vi "BMA Controller(No Promp).vi"() -> ()   [LabVIEW 2010]
uses:
  SubVIs/FP Buttons.llb/Login Button__FP.ctl
  SubVIs/FP Buttons.llb/Diagnose Button__FP.ctl
  SubVIs/FP Buttons.llb/Exchange Button__FP.ctl
  SubVIs/FP Buttons.llb/Comments Button__FP.ctl
  SubVIs/Front Panel.llb/Reset.ctl
  SubVIs/General.llb/Time Control(System).ctl
  SubVIs/Front Panel.llb/Add Recipe__FP-BMA.ctl
  SubVIs/Front Panel.llb/Delete Recipe__FP-BMA.ctl
  SubVIs/Front Panel.llb/Define Recipe__FP-BMA.ctl
  SubVIs/Front Panel.llb/Operation__FP-BMA.ctl
  SubVIs/Front Panel.llb/Warnings__FP-BMA.ctl
  SubVIs/Front Panel.llb/Input__FP-BMA.ctl
  SubVIs/Front Panel.llb/Output__FP-BMA.ctl
  SubVIs/Front Panel.llb/PID Sets__FP-BMA.ctl
  SubVIs/Front Panel.llb/Cascade__FP-BMA.ctl
  SubVIs/Front Panel.llb/Current Step__FP-BMA.ctl
  SubVIs/Data Communication.llb/Plot Settings__DC-BMA.ctl
  SubVIs/FP Buttons.llb/Table Button(FTF)__FP.ctl
  SubVIs/FP Buttons.llb/Try Button__FP.ctl
  SubVIs/FP Buttons.llb/Print Button__FP.ctl
  SubVIs/FP Buttons.llb/Exit__FP.ctl
  SubVIs/Structure.llb/Queue Operation Mode__STR.ctl
  SubVIs/Structure.llb/Queues__STR.ctl
  SubVIs/Controller Communication.llb/F4 Controller Input Data Global Function Enumi.ctl
panel:
  out "Comm Status":string
  out "Exec Status":string
  in  "DataExchange":T1
  in  "Diagnose Comm":T2
  in  "Recipe":T3
  in  "Graph View":T4
  in  "EventLog":T5
  in  "Print":T6
  in  "Exit":T7
  in  "Login":T8
  in  "Tab":T9(tab)=enum."控制F4数据交换"
  in  "COM Diags":i32(listbox)
  in  "Reset Statistics":T10
  in  "Time Elapsed":string
  in  "Time Window":i32 caption="时间窗"
  in  "Time Schedule":T11(ring)
  in  "Modify":T12
  in  "Delete":T13
  in  "Add":T14
  in  "Recipe Name":u16(ring) caption="Recipe名称"
  in  "Recipe Start Time":T15 format="%<%.3X %x>T"
  in  "Calenda Schedule":i32(listbox)
  in  "Schedule Strings":string="2009-04-30 时间表"
  out "Event Strings":string
  in  "Plot Scroll":i32(c297)
  in  "Plot Settings":T16[](array[typedef]) caption="曲线设置"
  out "Trend Plot":waveform(dbl)(graph)
  in  "开始时间":T15 format="%<%.3X %x>T"
  in  "Duration":cluster{"Days":dbl, "Hrs":dbl, "Mins":dbl} caption="持续时间"
  in  "F4 Operation":T24={"operation"=TRUE, "Alarms"=FALSE, "Inputs"=FALSE, "Outputs"=FALSE, "PID Sets"=FALSE, "cascade"=FALSE, "Current Step"=FALSE} caption="F4操作"
  # "环境试验箱控制系统"
  # "重置后的时间消耗"
  # "估计时间窗"
  # "设置recipe开始时间"
  # "设置Recipe名称"
  # "时间表"
  # "显示   控制器                参数类型                 参数                    索引                    轴"
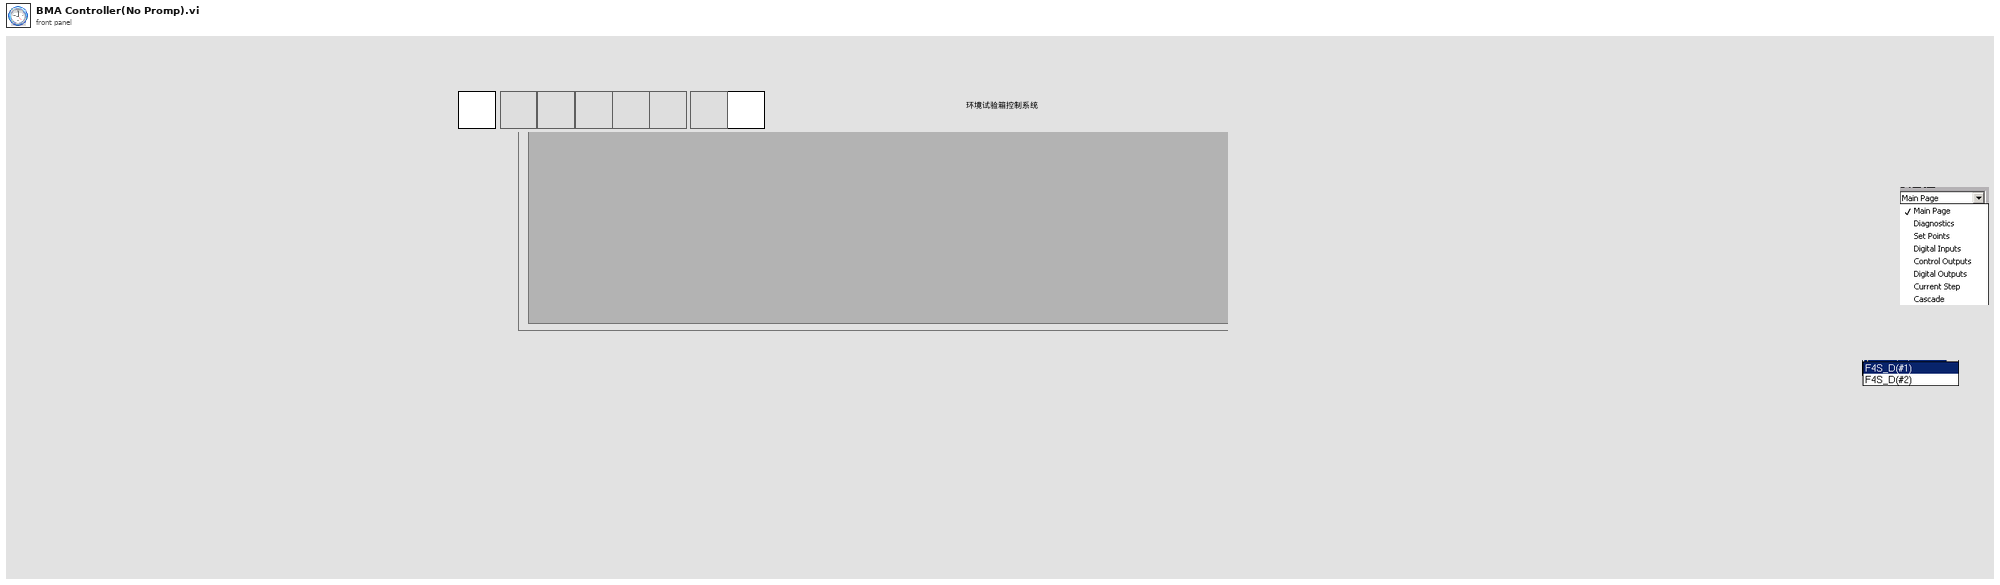
[diagram p1: front panel]
types:
  T1 = typedef "Try Button__FP.ctl" = bool
  T2 = typedef "Diagnose Button__FP.ctl" = bool
  T3 = typedef "Exchange Button__FP.ctl" = bool
  T4 = typedef "Table Button(FTF)__FP.ctl" = bool
  T5 = typedef "Comments Button__FP.ctl" = bool
  T6 = typedef "Print Button__FP.ctl" = bool
  T7 = typedef "Exit__FP.ctl" = bool
  T8 = typedef "Login Button__FP.ctl" = bool
  T9 = enum32{"通信诊断", "设置时间信息", "查看事件记录", "查看趋势图", "控制F4数据交换"}
  T10 = typedef "Reset.ctl" = bool
  T11 = enum16{"仅一次", "每隔数天", "每一天", "每个工作日", "每个周末", "每个月中的一天"}
  T12 = typedef "Define Recipe__FP-BMA.ctl" = bool
  T13 = typedef "Delete Recipe__FP-BMA.ctl" = bool
  T14 = typedef "Add Recipe__FP-BMA.ctl" = bool
  T15 = typedef "Time Control(System).ctl" = timestamp
  T16 = typedef "Plot Settings__DC-BMA.ctl" = cluster{"Show?":bool, "Controller Type":enum16{"F4S_D(#1)", "F4S_D(#2)"}, "Parameter":enum16{"主要页面", "诊断", "设置点", "数字输入", "控制输出", "数字输出", "当前步骤", "Cascade"}, "Parameter":enum16{"冷端补偿1", "冷端补偿2"}, "索引":enum16{"F4S_D(#1)"}, "Axis":string}
  T17 = typedef "Operation__FP-BMA.ctl" = bool
  T18 = typedef "Warnings__FP-BMA.ctl" = bool
  T19 = typedef "Input__FP-BMA.ctl" = bool
  T20 = typedef "Output__FP-BMA.ctl" = bool
  T21 = typedef "PID Sets__FP-BMA.ctl" = bool
  T22 = typedef "Cascade__FP-BMA.ctl" = bool
  T23 = typedef "Current Step__FP-BMA.ctl" = bool
  T24 = cluster{"operation":T17, "Alarms":T18, "Inputs":T19, "Outputs":T20, "PID Sets":T21, "cascade":T22, "Current Step":T23}
  T25 = typedef "Queue Operation Mode__STR.ctl" = enum16{"Noop", "Send Main", "Send Process", "Flush", "Destroy"}
  T26 = typedef "Queues__STR.ctl" = cluster{"main":T27, "process bar":T27}
  T27 = typedef "Queue RefNum" = refnum<k1>
  T28 = cluster{"[0]":bool, "[1]":bool, "[2]":bool, "[3]":bool, "[4]":bool, "[5]":bool, "[6]":bool}
  T29 = enum32{"Invalid", "Standard", "Closed", "Hidden", "Minimized", "Maximized"}
  T30 = enum32{"invalid app kind", "Development System", "Run Time System", "Student Edition", "Embedded LabVIEW", "Evaluation", "Custom"}
  T31 = typedef "F4 Controller Input Data Global Function Enumi.ctl" = enum16{"保存数据", "读取数据", "主程序状态写入", "主程序状态读取"}
  T32 = cluster{"Core":cluster{"Current VI Reference":refnum<vi>, "Close Panel on Exit?":bool}, "queues":T26, "Menu Refnum":refnum<k9>, "button":refnum<vi>[], "Tab":enum32{"通信诊断", "设置时间信息", "查看事件记录", "查看趋势图", "控制F4数据交换"}}
  T33 = cluster{"Current VI Reference":refnum<vi>, "Close Panel on Exit?":bool}
  T34 = typedef "Path InitPaths__FS.ctl" = cluster{"Ctrller CFG":path, "INI":path, "Profile":path, "EventLog":path, "Data":path}
  T35 = typedef "Controller Configuration__CHC.ctl" = cluster{"Ctrller Type":T36, "Ctrller Name":string, "Ctrller Addr":string, "Server IP":string, "Conn Result":string, "Port":string, "Baud":dbl}
  T36 = typedef "Controller Configuration__Ctrller Type.ctl" = enum16{"F4S/D", "Synergy"}
  T37 = typedef "Login Info__BMA-ULR.ctl" = cluster{"status":bool, "account":u16, "user":string}
  T38 = cluster{"Plot Settings":refnum<vi>, "Plot Scroll":refnum<vi>}
  T39 = typedef "Path InitDynamicVIsPaths__FS.ctl" = cluster{"F4 Operation":path, "F4 Alarms":path, "F4 Inputs":path, "F4 Outputs":path, "F4 PID Sets":path, "F4 Cascade":path, "F4 Current Step":path, "Profile SubPanel":path, "Profile Editor":path, "MainVI":path, "Profile Control":path, "Synergy Control":path, "Driver Server":path}
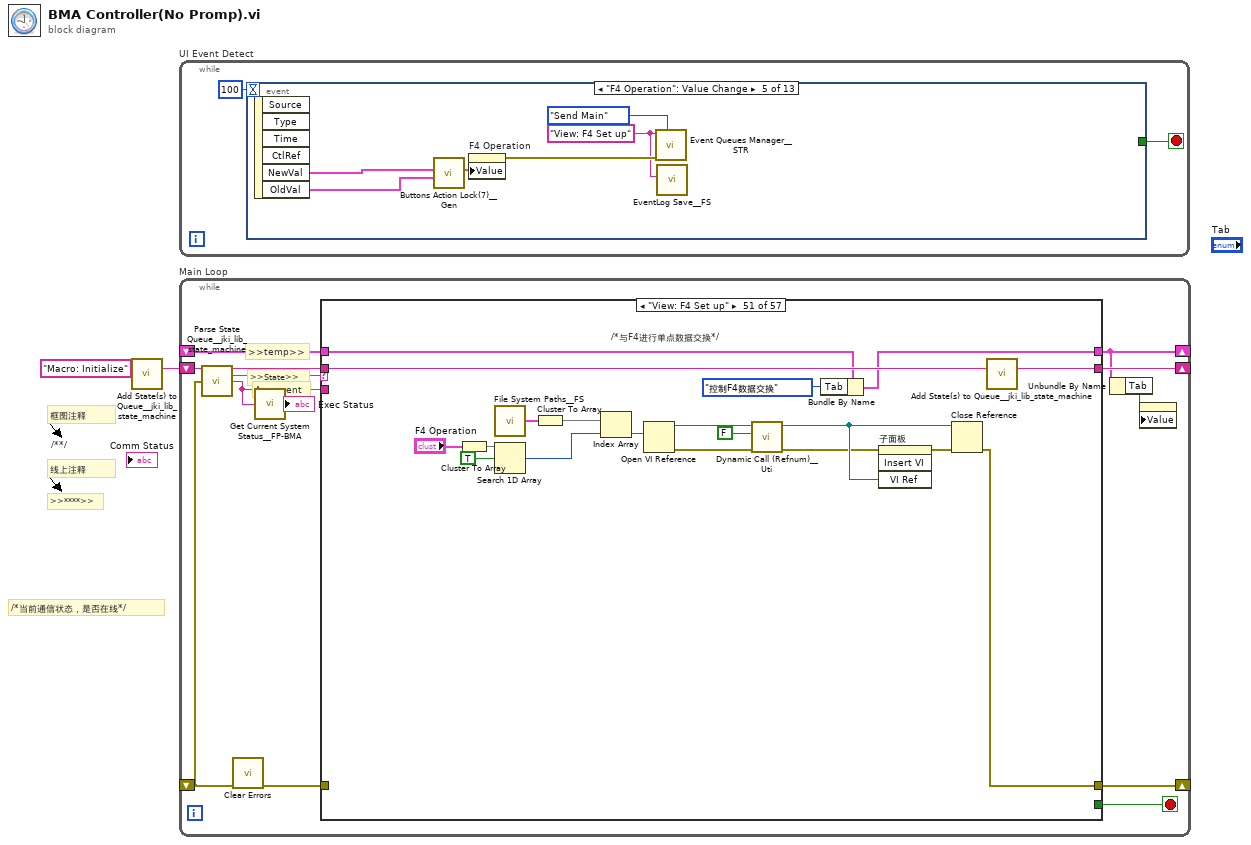
[diagram p0: block diagram]
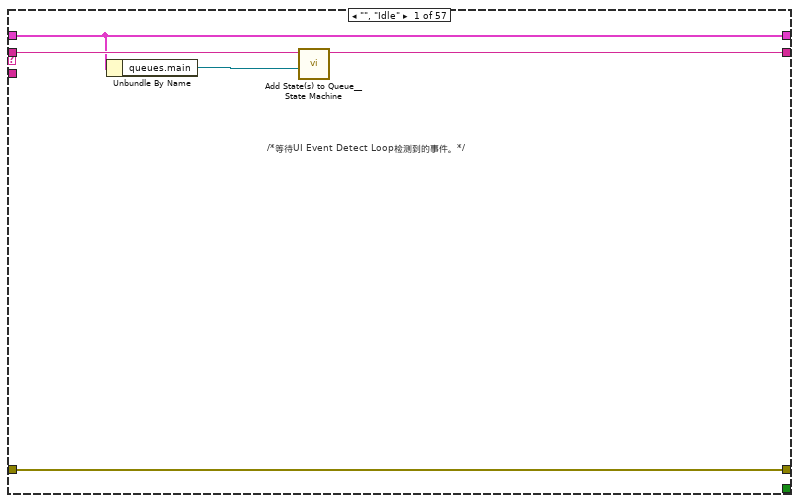
[diagram p2: hidden frame]
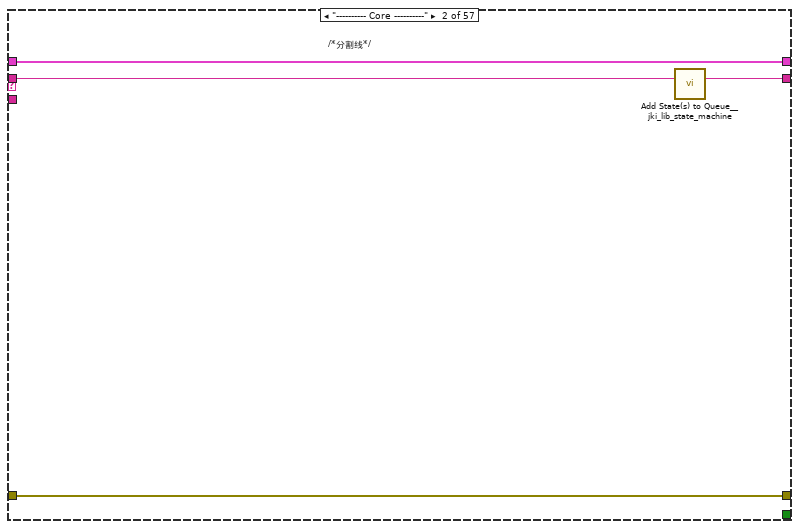
[diagram p3: hidden frame]
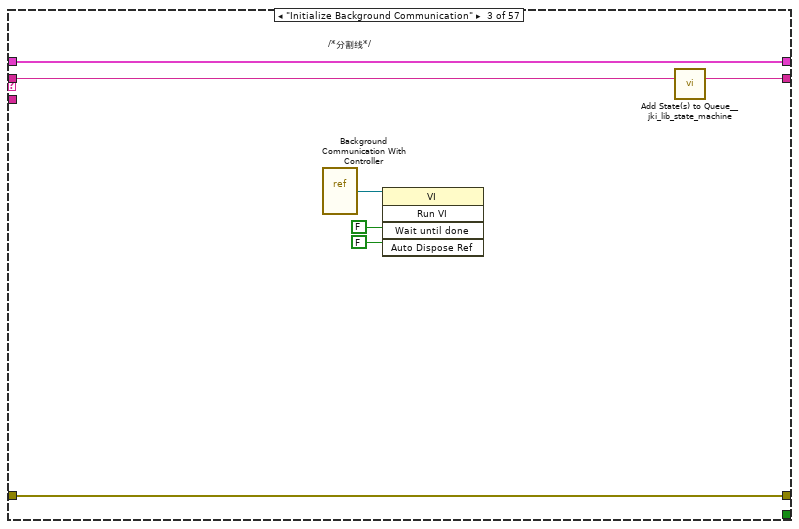
[diagram p4: hidden frame]
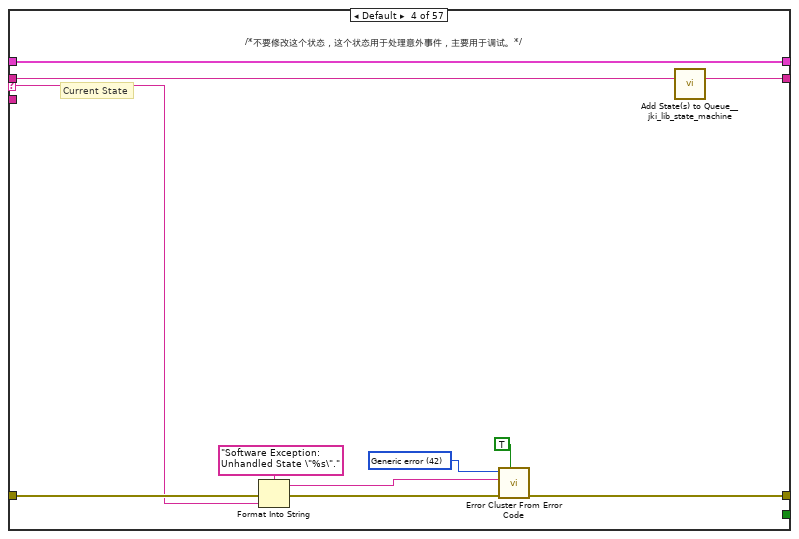
[diagram p5: hidden frame]
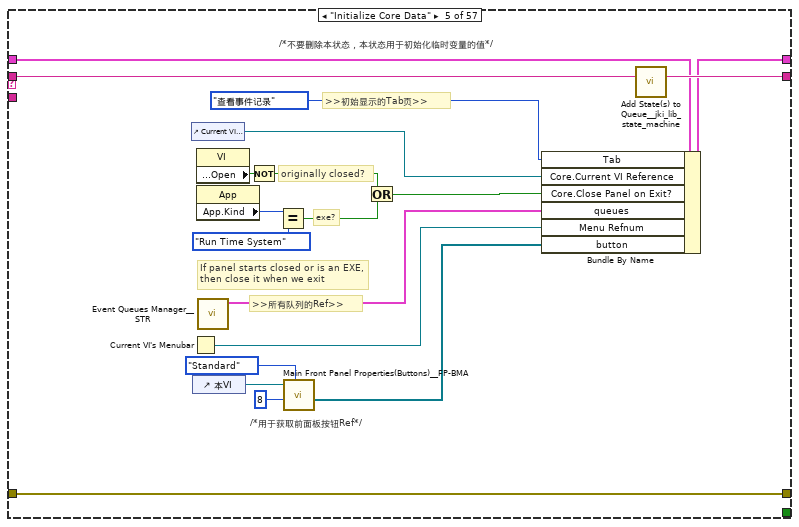
[diagram p6: hidden frame]
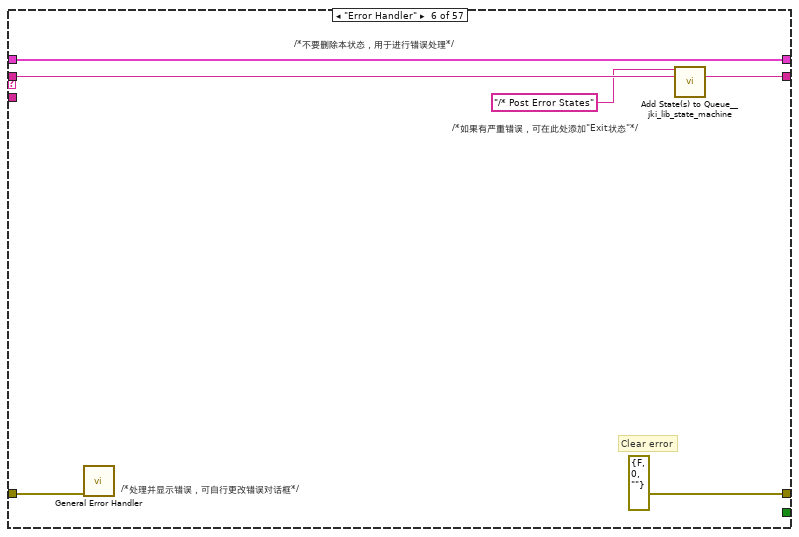
[diagram p7: hidden frame]
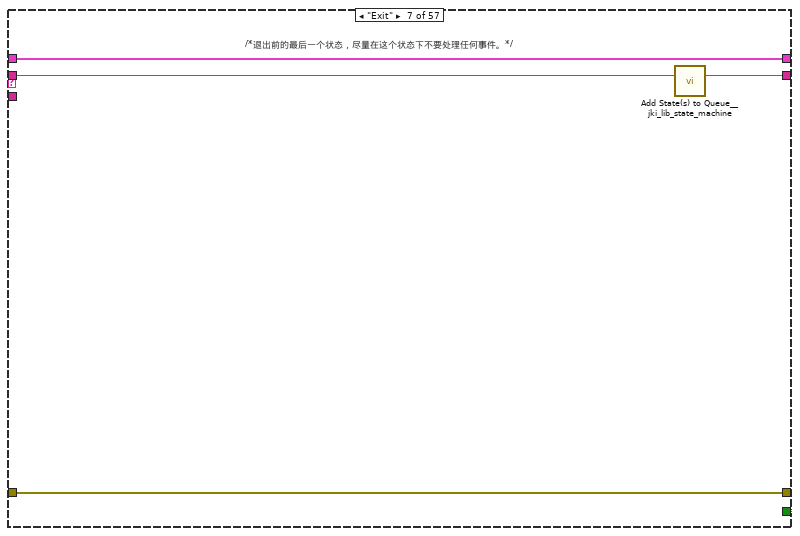
[diagram p8: hidden frame]
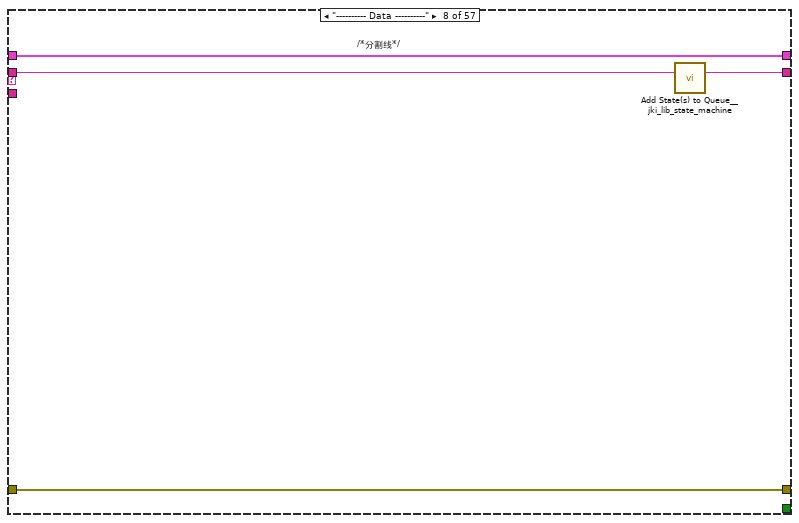
[diagram p9: hidden frame]
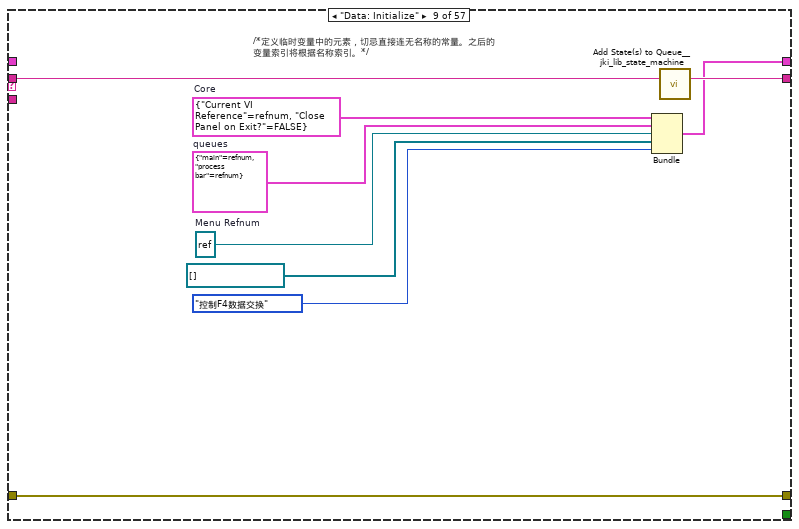
[diagram p10: hidden frame]
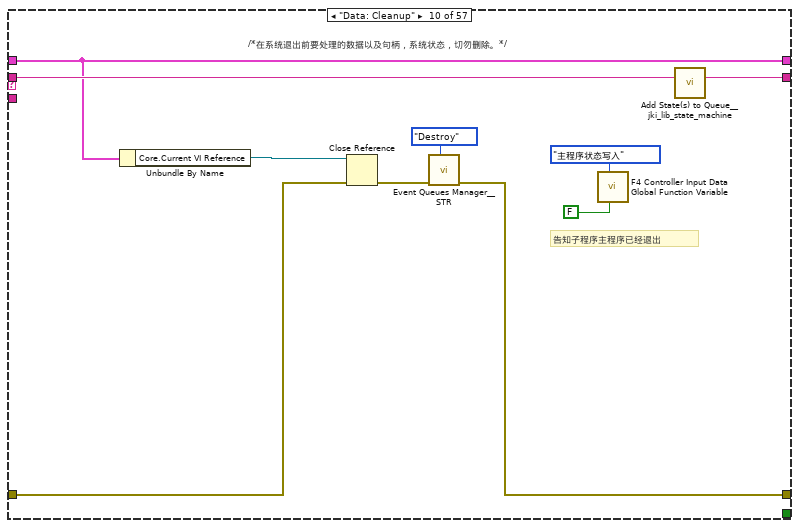
[diagram p11: hidden frame]
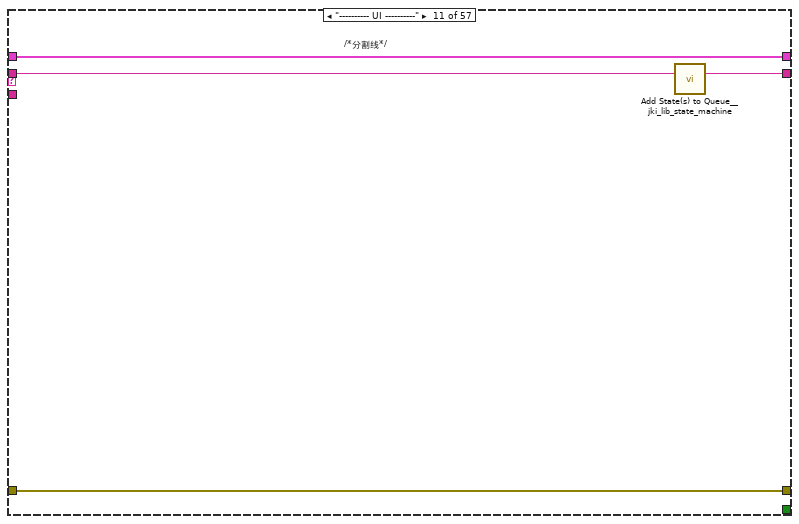
[diagram p12: hidden frame]
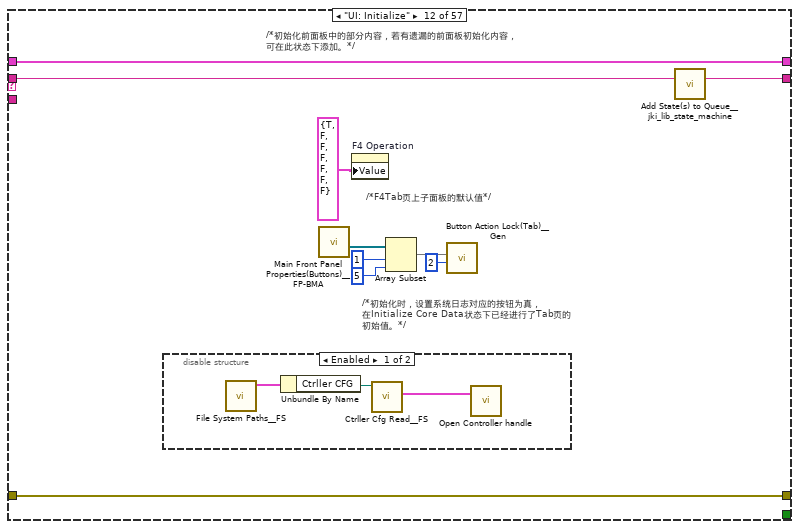
[diagram p13: hidden frame]
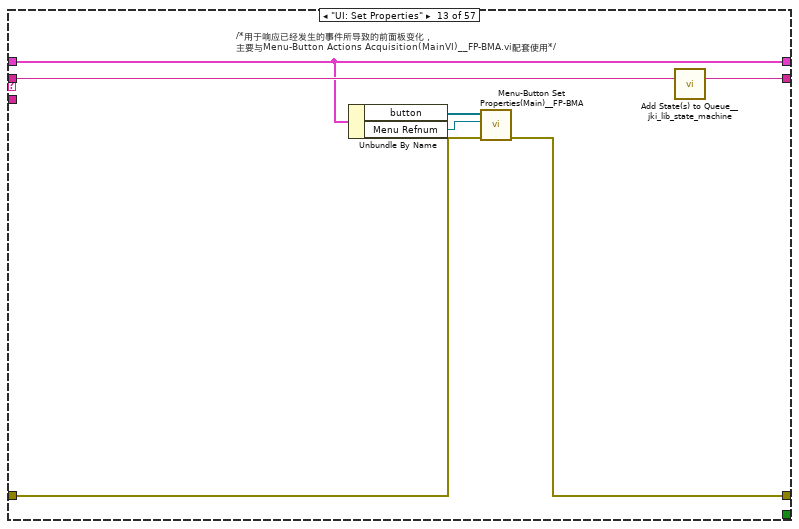
[diagram p15: hidden frame]
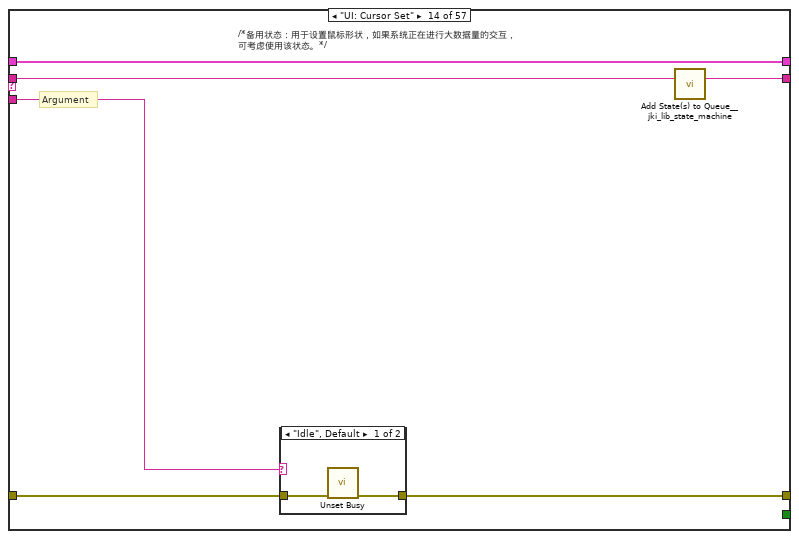
[diagram p16: hidden frame]
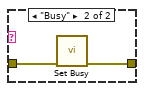
[diagram p17: hidden frame]
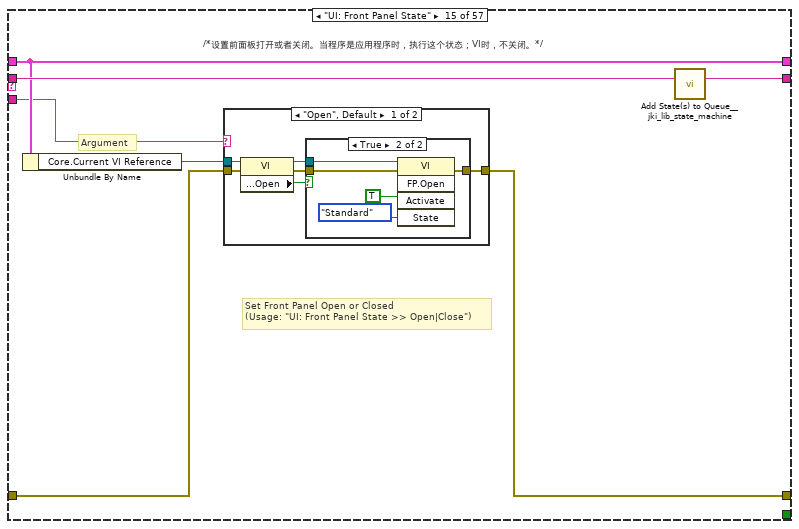
[diagram p18: hidden frame]
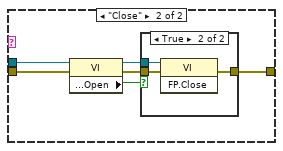
[diagram p20: hidden frame]
diagram:
  # "/**/"
  # "框图注释"
  # "线上注释"
  # ">>****>>"
  # "/*当前通信状态，是否在线*/"
  n1 = call "Add State(s) to Queue__jki_lib_state_machine.vi"("State(s) in (\"\")"="Macro: Initialize") -> ("States Out"=w1:string)  [unwired: 14 in]
  n2 = while "UI Event Detect" {
    stop <- w3 stop-if-true
    n3 = event shown="[4] \"F4 Operation\": Value Change" {
      selector: _ -> [_ _ _ _ _ _ _ _ _ _ _ _ _]
      dyn-events: _ -> [_ _ _ _ _ _ _ _ _ _ _ _ _]
      timeout: 100 -> [_ _ _ _ _ _ _ _ _ _ _ _ _]
      tunnel: [w5 _ _ _ _ _ _ _ _ _ _ _ _] -> w3
      event Timeout {
        n4 = event-data() -> ()  [unwired: 1 in, 2 out]
        n5 = call "Event Queues Manager__STR.vi"("mode"=Queue_Operation_Mode__STR."Noop") -> ("queues out"=w7:T26)  [unwired: 9 in, 1 out]
        n6 = Unbundle By Name(w7) -> ("main"=w6:T27)
        n7 = call <vilib>:"Not A Queue.vi"("queue"=w6) -> ("is a queue?"=w5:bool)
      }
      event Menu Selection (User) {
        n8 = event-data() -> ("ItemTag"=w9:string, "MenuRef"=w10:refnum<k9>)  [unwired: 1 in, 3 out]
        n9 = call "EventLog Save__FS.vi"("Event"=w9) -> ()  [unwired: 10 in, 1 out]
        n10 = call "Menu Get Event Message__FP-BMA.vi"("menu ref in"=w10, "menu item in"=w9) -> ("message"=w11:variant, "menu item out"=w12:string, "mode"=w13:T25)  [unwired: 7 in]
        n11 = call "Event Queues Manager__STR.vi"("mode"=w13, "message"=w11, "event"=w12) -> ()  [unwired: 7 in, 2 out]
      }
      event Value Change {
        w14 = "Macro: Exit"
        n12 = event-data() -> ()  [unwired: 1 in, 5 out]
        n13 = call "Event Queues Manager__STR.vi"("mode"=Queue_Operation_Mode__STR."Send Main", "event"=w14) -> ()  [unwired: 8 in, 2 out]
        n14 = call "EventLog Save__FS.vi"("Event"=w14) -> ()  [unwired: 10 in, 1 out]
      }
      event Panel Close? {
        w16 = "Macro: Exit"
        n15 = event-data() -> ()  [unwired: 1 in, 4 out]
        n16 = call "Event Queues Manager__STR.vi"("mode"=Queue_Operation_Mode__STR."Send Main", "event"=w16) -> ()  [unwired: 8 in, 2 out]
        n17 = call "EventLog Save__FS.vi"("Event"=w16) -> ()  [unwired: 10 in, 1 out]
        n18 = event-data("Discard?"=TRUE ("放弃？")) -> ()  [unwired: 1 in, 1 out]
      }
      event "F4 Operation": Value Change {
        w19 = "View: F4 Set up"
        n19 = event-data() -> ("NewVal"=w23:T24, "OldVal"=w22:T24)  [unwired: 1 in, 4 out]
        n20 = call "Buttons Action Lock(7)__Gen.vi"("Original Value"=w22, "New Value In"=w23) -> ("New Value Out"=w20:T28)  [unwired: 9 in]
        n21 = property on="F4 Operation" class="Clust (strict)"("Value"=w20) -> (error out=w21:errorcluster)  [unwired: 2 in, 1 out]
        n22 = call "Event Queues Manager__STR.vi"("mode"=Queue_Operation_Mode__STR."Send Main", "error in (no error)"=w21, "event"=w19) -> ()  [unwired: 7 in, 2 out]
        n23 = call "EventLog Save__FS.vi"("Event"=w19) -> ()  [unwired: 10 in, 1 out]
      }
      event "Plot Scroll": Value Change {
        n24 = event-data() -> ()  [unwired: 1 in, 6 out]
        n25 = Build Array("Plot Scroll") -> (w25:i32[])
        n26 = property on="Plot Settings" class="Arr (strict)"("Index Values"=w25) -> ()  [unwired: 2 in, 2 out]
      }
      event Value Change {
        w27 = "Users: Login"
        n27 = event-data() -> ()  [unwired: 1 in, 6 out]
        n28 = call "Event Queues Manager__STR.vi"("mode"=Queue_Operation_Mode__STR."Send Main", "message"="Login", "event"=w27) -> ()  [unwired: 7 in, 2 out]
        n29 = call "EventLog Save__FS.vi"("Event"=w27) -> ()  [unwired: 10 in, 1 out]
      }
      event Value Change {
        w35 = "System: Comm Diags"
        n30 = event-data() -> ()  [unwired: 1 in, 6 out]
        n31 = call "Main Front Panel Properties(Buttons)__FP-BMA.vi"() -> ("button"=w34:refnum<vi>[])  [unwired: 6 in, 5 out]
        n32 = Array Subset(array=w34, index=1 ("索引"), length=5 ("长度")) -> (w31:refnum<vi>[])
        n33 = call "Button Action Lock(Tab)__Gen.vi"("Index(T)"=0, "Tab Action"=w31) -> ()  [unwired: 10 in]
        n34 = call "Event Queues Manager__STR.vi"("mode"=Queue_Operation_Mode__STR."Send Main", "event"=w35) -> ()  [unwired: 8 in, 2 out]
        n35 = call "EventLog Save__FS.vi"("Event"=w35) -> ()  [unwired: 10 in, 1 out]
      }
      event Value Change {
        w42 = "View: Synergy Set up"
        n36 = event-data() -> ()  [unwired: 1 in, 6 out]
        n37 = call "Main Front Panel Properties(Buttons)__FP-BMA.vi"() -> ("button"=w41:refnum<vi>[])  [unwired: 6 in, 5 out]
        n38 = Array Subset(array=w41, index=1 ("索引"), length=5 ("长度")) -> (w38:refnum<vi>[])
        n39 = call "Button Action Lock(Tab)__Gen.vi"("Index(T)"=1, "Tab Action"=w38) -> ()  [unwired: 10 in]
        n40 = call "Event Queues Manager__STR.vi"("mode"=Queue_Operation_Mode__STR."Send Main", "event"=w42) -> ()  [unwired: 8 in, 2 out]
        n41 = call "EventLog Save__FS.vi"("Event"=w42) -> ()  [unwired: 10 in, 1 out]
      }
      event Value Change {
        w49 = "EventLogs: View"
        n42 = event-data() -> ()  [unwired: 1 in, 6 out]
        n43 = call "Main Front Panel Properties(Buttons)__FP-BMA.vi"() -> ("button"=w48:refnum<vi>[])  [unwired: 6 in, 5 out]
        n44 = Array Subset(array=w48, index=1 ("索引"), length=5 ("长度")) -> (w45:refnum<vi>[])
        n45 = call "Button Action Lock(Tab)__Gen.vi"("Index(T)"=2, "Tab Action"=w45) -> ()  [unwired: 10 in]
        n46 = call "EventLog Save__FS.vi"("Event"=w49) -> ()  [unwired: 10 in, 1 out]
        n47 = call "Event Queues Manager__STR.vi"("mode"=Queue_Operation_Mode__STR."Send Main", "event"=w49) -> ()  [unwired: 8 in, 2 out]
      }
      event Value Change {
        w56 = "TP: Graph"
        n48 = event-data() -> ()  [unwired: 1 in, 6 out]
        n49 = call "Main Front Panel Properties(Buttons)__FP-BMA.vi"() -> ("button"=w55:refnum<vi>[])  [unwired: 6 in, 5 out]
        n50 = Array Subset(array=w55, index=1 ("索引"), length=5 ("长度")) -> (w52:refnum<vi>[])
        n51 = call "Button Action Lock(Tab)__Gen.vi"("Index(T)"=3, "Tab Action"=w52) -> ()  [unwired: 10 in]
        n52 = call "EventLog Save__FS.vi"("Event"=w56) -> ()  [unwired: 10 in, 1 out]
        n53 = call "Event Queues Manager__STR.vi"("mode"=Queue_Operation_Mode__STR."Send Main", "event"=w56) -> ()  [unwired: 8 in, 2 out]
      }
      event Value Change {
        w63 = "View: F4 Set up"
        n54 = event-data() -> ()  [unwired: 1 in, 6 out]
        n55 = call "Main Front Panel Properties(Buttons)__FP-BMA.vi"() -> ("button"=w62:refnum<vi>[])  [unwired: 6 in, 5 out]
        n56 = Array Subset(array=w62, index=1 ("索引"), length=5 ("长度")) -> (w59:refnum<vi>[])
        n57 = call "Button Action Lock(Tab)__Gen.vi"("Index(T)"=4, "Tab Action"=w59) -> ()  [unwired: 10 in]
        n58 = call "Event Queues Manager__STR.vi"("mode"=Queue_Operation_Mode__STR."Send Main", "event"=w63) -> ()  [unwired: 8 in, 2 out]
        n59 = call "EventLog Save__FS.vi"("Event"=w63) -> ()  [unwired: 10 in, 1 out]
      }
      event Value Change {
        w65 = "File: Print"
        n60 = event-data() -> ()  [unwired: 1 in, 6 out]
        n61 = call "Event Queues Manager__STR.vi"("mode"=Queue_Operation_Mode__STR."Send Main", "event"=w65) -> ()  [unwired: 8 in, 2 out]
        n62 = call "EventLog Save__FS.vi"("Event"=w65) -> ()  [unwired: 10 in, 1 out]
      }
    }
  }
  n63 = while "Main Loop" {
    shift-right: [w71] -> _
    shift-left: _ -> [w74]
    shift-right: [w77] -> _
    shift-left: _ -> [w72]
    shift-right: [w76] -> _
    shift-left: w1 -> [w78]
    stop <- w75 stop-if-true
    # "Argument"
    # ">>State>>"
    # ">>temp>>"
    n64 = call "Parse State Queue__jki_lib_state_machine.vi"("State Queue"=w78, "Error In (no error)"=w72) -> ("Remaining States"=w79:string, "Current State"=w73:string, "Arguments"=w68:string)  [unwired: 11 in]
    n65 = call <vilib>:"Clear Errors.vi"("error in (no error)"=w72) -> ("error out"=w67:errorcluster)  [unwired: 6 in]
    n66 = call "Get Current System Status__FP-BMA.vi"("current state"=w68) -> ("system status"=→"Exec Status":string)
    n67 = case shown="\"View: F4 Set up\"" w73 {
      selector: w73 -> [_ _ _ w96 _ _ _ _ _ _ _ _ _ _ _ _ _ _ _ _ _ _ _ _ _ _ _ _ _ _ _ _ _ _ _ _ _ _ _ _ _ _ _ _ _ _ _ _ _ _ _ _ _ _ _ _ _]
      tunnel: w79 -> [w84 w88 w95 w100 w125 w131 w136 w140 w149 w159 w163 w173 w183 w189 w200 w226 w231 w241 w242 w249 w261 w286 w290 w294 w298 w302 w306 w311 w315 w319 w323 w329 w333 w337 w341 w345 w349 w353 w357 w363 w367 w371 w379 w383 w387 w391 w403 w407 w411 w415 w434 w443 w447 w451 w455 w464 w474]
      tunnel: w68 -> [_ _ _ _ _ _ _ _ _ _ _ _ _ w184 w194 _ _ _ _ _ _ _ _ _ _ _ _ _ _ _ _ _ _ _ _ _ _ _ _ _ _ _ _ _ _ _ _ _ _ _ _ _ _ _ _ _ _]
      tunnel: w74 -> [w83 w85 w92 w98 w116 w128 w134 w137 _ w155 w160 w171 w179 w187 w196 w223 w228 w238 w243 w246 w254 w283 w287 w291 w295 w299 w303 w308 w312 w316 w320 w325 w330 w334 w338 w342 w346 w350 w354 w360 w364 w368 w374 w380 w384 w388 w400 w404 w408 w412 w422 w441 w444 w448 w452 w462 w472]
      tunnel: [w80 w86 w93 w102 w122 errorcluster {"status"=FALSE, "code"=0, "source"=""} ("error out") w133 w138 w146 w152 w161 w170 w177 w185 w197 w224 w229 w239 w244 w247 w251 w284 w288 w292 w296 w300 w304 w309 w313 w317 w321 w327 w331 w335 w339 w343 w347 w351 w355 w361 w365 w369 w375 w381 w385 w389 w401 w405 w409 w413 w421 w436 w445 w449 w453 w456 w467] -> w77
      tunnel: w67 -> [w80 w86 w93 w101 w122 w127 w133 w138 w146 w156 w161 w170 w178 w186 w198 w224 w229 w239 w244 w247 w252 w284 w288 w292 w296 w300 w304 w309 w313 w317 w321 w327 w331 w335 w339 w343 w347 w351 w355 w361 w365 w369 w376 w381 w385 w389 w401 w405 w409 w413 _ w435 w445 w449 w453 w457 w466]
      tunnel: [w82 w87 w94 w99 w124 w130 w135 w139 w148 w158 w162 w172 w182 w188 w199 w225 w230 w240 w242 w248 w260 w285 w289 w293 w297 w301 w305 w310 w314 w318 w322 w328 w332 w336 w340 w344 w348 w352 w356 w362 w366 w370 w378 w382 w386 w390 w402 w406 w410 w414 w433 w442 w446 w450 w454 w463 w473] -> w76
      tunnel: [_ _ _ _ _ _ TRUE _ _ _ _ _ _ _ _ _ _ _ _ _ _ _ _ _ _ _ _ _ _ _ _ _ _ _ _ _ _ _ _ _ _ _ _ _ _ _ _ _ _ _ _ _ _ _ _ _ _] -> w75
      tunnel: [w83 w85 w92 w98 w123 w128 w134 w137 w147 w155 w160 w171 w179 w187 w196 w223 w228 w238 w243 w246 w254 w283 w287 w291 w295 w299 w303 w308 w312 w316 w320 w324 w330 w334 w338 w342 w346 w350 w354 w359 w364 w368 w373 w380 w384 w388 w399 w404 w408 w412 w424 w441 w444 w448 w452 w462 w472] -> w71
      frame "", "Idle" {
        # "/*等待UI Event Detect Loop检测到的事件。*/"
        n68 = Unbundle By Name(w83) -> ("queues.main"=w81:T27)
        n69 = call "Add State(s) to Queue__State Machine.vi"("queue"=w81, "State(s) in (\"\")"=w84) -> ("States Out"=w82:string)  [unwired: 8 in, 1 out]
      }
      frame "---------- Core ----------" {
        # "/*分割线*/"
        n70 = call "Add State(s) to Queue__jki_lib_state_machine.vi"("State(s) in (\"\")"=w88) -> ("States Out"=w87:string)  [unwired: 14 in]
      }
      frame "Initialize Background Communication" {
        # "/*分割线*/"
        n71 = vi-ref "Background Communication With Controller.vi"() -> (w91:refnum<vi>)
        n72 = invoke class="VI" method="Run VI"(reference=w91, "Wait until done"=FALSE ("结束前等待"), "Auto Dispose Ref"=FALSE ("自动销毁引用")) -> ()  [unwired: 2 in, 5 out]
        n73 = call "Add State(s) to Queue__jki_lib_state_machine.vi"("State(s) in (\"\")"=w95) -> ("States Out"=w94:string)  [unwired: 14 in]
      }
      frame Default {
        w105 = 42 items=["No error", "Argument error", "Memory is full", "Out of zone", "End of file", "File already open", "Generic file I/O error", "File not found", "File permission error", "Disk is full", "Duplicate path", "Too many files open", "System feature not enabled", "Resource file not found", "Cannot add resource", "Resource not found", "Image not found", "Image memory error", "Pen does not exist", "Config type invalid", "Config token not found", "Config parse error", "Config memory error", "Bad external code format", "Bad external code offset", "External code not present", "Null window", "Destroy window error", "Null menu", "Print aborted", "Bad print record", "Print driver error", "Windows error during printing", "Memory error during printing", "Print dialog error", "Generic print error", "Invalid device refnum", "Device not found", "Device parameter error", "Device unit error", "Cannot open device", "Device call aborted", "Generic error", "Cancelled by user", "Object ID too low", "Object ID too high", "Object not in heap", "Unknown heap", "Unknown object (invalid DefProc)", "Unknown object (DefProc not in table)", "Message out of range", "Invalid (null) method", "Unknown message", "Manager call not supported", "Bad address", "Network operation in progress", "Network operation timed out", "Connection is busy", "Network attribute not supported", "Network error", "Address in use", "System out of memory", "Connection aborted", "Connection refused", "Not connected", "Already connected", "Connection closed", "Initialization error (interapplication manager)", "Bad occurrence", "Wait on unbound occurrence handler", "Occurrence queue overflow", "Datalog type conflict", "Unused", "Unrecognized type (interapplication manager)", "Memory corrupt", "Failed to make temporary DLL", "Old CIN version", "Drag socket not found", "Failed to load drop-object", "Failed to register OLE object", "Failed to release OLE object", "Format specifier type mismatch", "Unknown format specifier", "Too few format specifiers", "Too many format specifiers", "Scan failed", "Newer CIN version", "Error converting to variant", "Runtime menu error", "Password tampered", "Variant attribute not found", "Incompatible variant data type", "Event data is not available", "Event Store is not present", "Occurrence is not found", "Event Queue is not created", "Event info is not available", "Refnum passed is NULL", "Error retrieving Class GUID", "Error retrieving CoClass GUID", "Error retrieving TypeLib GUID.", "Bad built application magic bytes.", "Specific driver is different from the specific driver associated with the Logical Name.", "There is no session opened to the class driver.", "Max Error", "MAX - Error with config objects", "MAX - Error loading configuration", "MAX - Group not supported"]
        # "/*不要修改这个状态，这个状态用于处理意外事件，主要用于调试。*/"
        # "Current State"
        n74 = Format Into String(format string="Software Exception: Unhandled State \"%s\"." ("message"), error in=w101, w96) -> (resulting string=w104:string, error out=w103:errorcluster)  [unwired: 1 in]
        n75 = call <vilib>:"Error Cluster From Error Code.vi"("show call chain? (False)"=TRUE, "error in (no error)"=w103, "error message (\"\")"=w104, "error code (0)"=w105) -> ("error out"=w102:errorcluster)  [unwired: 5 in]
        n76 = call "Add State(s) to Queue__jki_lib_state_machine.vi"("State(s) in (\"\")"=w100) -> ("States Out"=w99:string)  [unwired: 14 in]
      }
      frame "Initialize Core Data" {
        # ">>初始显示的Tab页>>"
        # ">>所有队列的Ref>>"
        # "/*用于获取前面板按钮Ref*/"
        # "/*不要删除本状态，本状态用于初始化临时变量的值*/"
        # "originally closed?"
        # "exe?"
        # "If panel starts closed or is an EXE, then close it when we exit"
        n77 = Current VI's Menubar() -> (w112:refnum<k9>)
        n78 = control-ref of="Current VI Reference"() -> (w114:refnum<vi>)
        n79 = control-ref of="本VI"() -> (w110:refnum<vi>)
        n80 = property class="VI"() -> ("Front Panel.Open"=w121:bool)  [unwired: 2 in, 2 out]
        n81 = property class="App"() -> ("App.Kind"=w120:T30)  [unwired: 2 in, 2 out]
        n82 = call "Event Queues Manager__STR.vi"() -> ("queues out"=w113:T26)  [unwired: 10 in, 1 out]
        n83 = Not(x=w121) -> (.not. x?=w118:bool)
        n84 = Equal?(x=w120, y=T30."Run Time System" ("Application:Kind")) -> (x = y?=w117:bool)
        n85 = call "Main Front Panel Properties(Buttons)__FP-BMA.vi"("window state"=T29."Standard", "number of button"=8, "VI ref in"=w110) -> ("button"=w108:refnum<vi>[])  [unwired: 3 in, 5 out]
        n86 = Or(x=w118, y=w117) -> (x .or. y?=w115:bool)
        n87 = Bundle By Name(cluster=w116, "Tab"=T9."查看事件记录", "Core.Current VI Reference"=w114, "Core.Close Panel on Exit?"=w115, "queues"=w113, "Menu Refnum"=w112, "button"=w108) -> (w123:T32)
        n88 = call "Add State(s) to Queue__jki_lib_state_machine.vi"("State(s) in (\"\")"=w125) -> ("States Out"=w124:string)  [unwired: 14 in]
      }
      frame "Error Handler" {
        # "/*不要删除本状态，用于进行错误处理*/"
        # "/*如果有严重错误，可在此处添加\"Exit状态\"*/"
        # "/*处理并显示错误，可自行更改错误对话框*/"
        # "Clear error"
        n89 = call <vilib>:"General Error Handler.vi"("error in (no error)"=w127) -> ()  [unwired: 10 in, 5 out]
        n90 = call "Add State(s) to Queue__jki_lib_state_machine.vi"("State(s) in Front (\"\")"="/* Post Error States", "State(s) in (\"\")"=w131) -> ("States Out"=w130:string)  [unwired: 13 in]
      }
      frame "Exit" {
        # "/*退出前的最后一个状态，尽量在这个状态下不要处理任何事件。*/"
        n91 = call "Add State(s) to Queue__jki_lib_state_machine.vi"("State(s) in (\"\")"=w136) -> ("States Out"=w135:string)  [unwired: 14 in]
      }
      frame "---------- Data ----------" {
        # "/*分割线*/"
        n92 = call "Add State(s) to Queue__jki_lib_state_machine.vi"("State(s) in (\"\")"=w140) -> ("States Out"=w139:string)  [unwired: 14 in]
      }
      frame "Data: Initialize" {
        w144 = T26 {"main"=refnum, "process bar"=refnum}  # queues
        w145 = T33 {"Current VI Reference"=refnum, "Close Panel on Exit?"=FALSE}  # Core
        w143 = refnum<k9> refnum  # Menu Refnum
        # "/*定义临时变量中的元素，切忌直接连无名称的常量。之后的\n变量索引将根据名称索引。*/"
        n93 = Bundle("Core"=w145, "queues"=w144, "Menu Refnum"=w143, "button"=refnum<vi>[] [], "Tab"=T9."控制F4数据交换") -> (w147:T32)  [unwired: 1 in]
        n94 = call "Add State(s) to Queue__jki_lib_state_machine.vi"("State(s) in (\"\")"=w149) -> ("States Out"=w148:string)  [unwired: 14 in]
      }
      frame "Data: Cleanup" {
        # "告知子程序主程序已经退出"
        # "/*在系统退出前要处理的数据以及句柄，系统状态，切勿删除。*/"
        n95 = Unbundle By Name(w155) -> ("Core.Current VI Reference"=w157:refnum<vi>)
        n96 = Close Reference(reference=w157, error in (no error)=w156) -> (error out=w153:errorcluster)
        n97 = call "Event Queues Manager__STR.vi"("mode"=Queue_Operation_Mode__STR."Destroy", "error in (no error)"=w153) -> ("error out"=w152:errorcluster)  [unwired: 8 in, 1 out]
        n98 = call "F4 Controller Input Data Global Function Variable.vi"("主程序运行状态"=FALSE, "功能选择"=F4_Controller_Input_Data_Global_Function_Enumi."主程序状态写入") -> ()  [unwired: 8 in, 2 out]
        n99 = call "Add State(s) to Queue__jki_lib_state_machine.vi"("State(s) in (\"\")"=w159) -> ("States Out"=w158:string)  [unwired: 14 in]
      }
      frame "---------- UI ----------" {
        # "/*分割线*/"
        n100 = call "Add State(s) to Queue__jki_lib_state_machine.vi"("State(s) in (\"\")"=w163) -> ("States Out"=w162:string)  [unwired: 14 in]
      }
      frame "UI: Initialize" {
        # "/*初始化时，设置系统日志对应的按钮为真，\n在Initialize Core Data状态下已经进行了Tab页的\n初始值。*/"
        # "/*F4Tab页上子面板的默认值*/"
        # "/*初始化前面板中的部分内容，若有遗漏的前面板初始化内容，\n可在此状态下添加。*/"
        n101 = disable-structure shown="Enabled" {
          frame Enabled {
            n102 = call "File System Paths__FS.vi"() -> ("FilePaths"=w175:T34)  [unwired: 9 in, 2 out]
            n103 = Unbundle By Name(w175) -> ("Ctrller CFG"=w174:path)
            n104 = call "Ctrller Cfg Read__FS.vi"("Path In"=w174) -> ("Ctrllers"=w176:T35[])  [unwired: 8 in, 2 out]
            n105 = call "Open Controller handle.vi"("Ctrllers"=w176) -> ()  [unwired: 2 in, 1 out]
          }
          frame Disabled {
          }
        }
        n106 = call "Main Front Panel Properties(Buttons)__FP-BMA.vi"() -> ("button"=w164:refnum<vi>[])  [unwired: 6 in, 5 out]
        n107 = property on="F4 Operation" class="Clust (strict)"("Value"=T24 {"operation"=TRUE, "Alarms"=FALSE, "Inputs"=FALSE, "Outputs"=FALSE, "PID Sets"=FALSE, "cascade"=FALSE, "Current Step"=FALSE} ("F4 Operation")) -> ()  [unwired: 2 in, 2 out]
        n108 = Array Subset(array=w164, index=1 ("索引"), length=5 ("长度")) -> (w167:refnum<vi>[])
        n109 = call "Button Action Lock(Tab)__Gen.vi"("Index(T)"=2, "Tab Action"=w167) -> ()  [unwired: 10 in]
        n110 = call "Add State(s) to Queue__jki_lib_state_machine.vi"("State(s) in (\"\")"=w173) -> ("States Out"=w172:string)  [unwired: 14 in]
      }
      frame "UI: Set Properties" {
        # "/*用于响应已经发生的事件所导致的前面板变化，\n主要与Menu-Button Actions Acquisition(MainVI)__FP-BMA.vi配套使用*/"
        n111 = Unbundle By Name(w179) -> ("button"=w181:refnum<vi>[], "Menu Refnum"=w180:refnum<k9>)
        n112 = call "Menu-Button Set Properties(Main)__FP-BMA.vi"("error in (no error)"=w178, "menubar in"=w180, "controls in"=w181) -> ("error out"=w177:errorcluster)  [unwired: 6 in, 2 out]
        n113 = call "Add State(s) to Queue__jki_lib_state_machine.vi"("State(s) in (\"\")"=w183) -> ("States Out"=w182:string)  [unwired: 14 in]
      }
      frame "UI: Cursor Set" {
        # "/*备用状态：用于设置鼠标形状，如果系统正在进行大数据量的交互，\n可考虑使用该状态。*/"
        # "Argument"
        n114 = case shown="\"Idle\", Default" w184 {
          tunnel: w186 -> [w191 w193]
          tunnel: [w190 w192] -> w185
          frame "Idle", Default {
            n115 = call <vilib>:"Unset Busy.vi"("error in (no error)"=w191) -> ("error out"=w190:errorcluster)  [unwired: 10 in]
          }
          frame "Busy" {
            n116 = call <vilib>:"Set Busy.vi"("error in (no error)"=w193) -> ("error out"=w192:errorcluster)  [unwired: 9 in, 1 out]
          }
        }
        n117 = call "Add State(s) to Queue__jki_lib_state_machine.vi"("State(s) in (\"\")"=w189) -> ("States Out"=w188:string)  [unwired: 14 in]
      }
      frame "UI: Front Panel State" {
        # "/*设置前面板打开或者关闭。当程序是应用程序时，执行这个状态；VI时，不关闭。*/"
        # "Argument"
        # "Set Front Panel Open or Closed\n(Usage: \"UI: Front Panel State >> Open|Close\")"
        n118 = Unbundle By Name(w196) -> ("Core.Current VI Reference"=w195:refnum<vi>)
        n119 = case shown="\"Open\", Default" w194 {
          tunnel: w198 -> [w204 w217]
          tunnel: [w206 w218] -> w197
          tunnel: w195 -> [w205 w215]
          frame "Open", Default {
            n120 = property class="VI"(reference=w205, error in=w204) -> (reference out=w202:refnum<vi>, error out=w203:errorcluster, "Front Panel.Open"=w201:bool)
            n121 = case shown="True" w201 {
              tunnel: [w207 w210] -> w206
              tunnel: w203 -> [w207 w209]
              tunnel: w202 -> [_ w208]
              frame False {
              }
              frame True {
                n122 = invoke class="VI" method="FP.Open"(reference=w208, error in=w209, "Activate"=TRUE, "State"=T29."Standard") -> (error out=w210:errorcluster)  [unwired: 1 in, 4 out]
              }
            }
          }
          frame "Close" {
            n123 = property class="VI"(reference=w215, error in=w217) -> (reference out=w214:refnum<vi>, error out=w216:errorcluster, "Front Panel.Open"=w213:bool)
            n124 = case shown="True" w213 {
              tunnel: [w219 w222] -> w218
              tunnel: w216 -> [w219 w221]
              tunnel: w214 -> [_ w220]
              frame False {
              }
              frame True {
                n125 = invoke class="VI" method="FP.Close"(reference=w220, error in=w221) -> (error out=w222:errorcluster)  [unwired: 1 in, 2 out]
              }
            }
          }
        }
        n126 = call "Add State(s) to Queue__jki_lib_state_machine.vi"("State(s) in (\"\")"=w200) -> ("States Out"=w199:string)  [unwired: 14 in]
      }
      frame "---------- Macro ----------" {
        # "/*分割线*/"
        n127 = call "Add State(s) to Queue__jki_lib_state_machine.vi"("State(s) in (\"\")"=w226) -> ("States Out"=w225:string)  [unwired: 14 in]
      }
      frame "Macro: Initialize" {
        (unwired) "Data: Initialize\nInitialize Core Data\nUsers: Login\nUI: Initialize\nUI: Front Panel State >> Open\nUI: Set Properties\nInitialize Background Communication\nEventLogs: View\n"
        # "/*当VI运行时，首先执行它，可加载多个状态*/"
        # "/*初始化数据类型。\n弹出登陆对话框\n根据登陆的用户类型来初始化前面板\n设置前面板为打开\n设置前面板属性\n默认界面是查看F4设置*/"
        n128 = call "Add State(s) to Queue__jki_lib_state_machine.vi"("State(s) in Front (\"\")"="Data: Initialize\nInitialize Core Data\nUsers: Login\nUI: Initialize\nUI: Front Panel State >> Open\nUI: Set Properties\nInitialize Background Communication\nEventLogs: View\n", "State(s) in (\"\")"=w231) -> ("States Out"=w230:string)  [unwired: 13 in]
      }
      frame "Macro: Exit" {
        # "/*控制退出*/"
        n129 = Unbundle By Name(w238) -> ("Core.Close Panel on Exit?"=w237:bool)
        n130 = Select(t="UI: Front Panel State >> Close", s=w237, f="") -> (s? t:f=w234:string)
        n131 = call "Add State(s) to Queue__jki_lib_state_machine.vi"("State(s) in (\"\")"=w234, "State(s) at Back (\"\")"="Data: Cleanup\nExit") -> ("States Out"=w232:string)  [unwired: 13 in]
        n132 = call "Add State(s) to Queue__jki_lib_state_machine.vi"("State(s) in Front (\"\")"=w232, "State(s) in (\"\")"=w241) -> ("States Out"=w240:string)  [unwired: 13 in]
      }
      frame "----------User Management ----------" {
        # "/*分割线*/"
      }
      frame "Users: Login" {
        # "/*定义用户登录时，接下来的状态*/"
        n133 = call "Add State(s) to Queue__jki_lib_state_machine.vi"("State(s) in Front (\"\")"="Users: Login Dialog\nUI: Set Properties", "State(s) in (\"\")"=w249) -> ("States Out"=w248:string)  [unwired: 13 in]
      }
      frame "Users: Login Dialog" {
        # "/*弹出登陆对话框，并根据用户级别定义前面板哪些功能使能。*/"
        n134 = First Call?() -> (First Call?: T/F=w250:bool)
        n135 = Unbundle By Name(w254) -> ("Menu Refnum"=w259:refnum<k9>)
        n136 = control-ref of="Login"() -> (w258:refnum<vi>)
        n137 = case shown="False" w250 {
          tunnel: w259 -> [w271 w276]
          tunnel: w258 -> [w270 w275]
          tunnel: [w265 FALSE ("failed at first login?")] -> w253
          tunnel: w252 -> [w263 _]
          tunnel: [w262 w280] -> w251
          frame False {
            # ">>用户级别>>"
            n138 = call "Login Info FGV__BMA-ULR.vi"() -> ("login info out"=w267:T37)  [unwired: 2 in]
            n139 = call "Dialog System Login__BMA-ULI.vi"("error in (no error)"=w263, "login info in"=w267) -> ("error out"=w264:errorcluster, "failed at first login?"=w265:bool, "login info out"=w266:T37)  [unwired: 7 in]
            n140 = call "Login Info FGV__BMA-ULR.vi"("login info in"=w266, "read/write (F:read)"=TRUE) -> ("login info out"=w272:T37)
            n141 = call "Login Menu Button Properties Update__BMA-FP.vi"("error in (no error)"=w264, "login button"=w270, "menubar in"=w271, "login info in"=w272) -> ("error out"=w269:errorcluster, "login info out"=w268:T37)  [unwired: 6 in]
            n142 = call "Menu-Button Get User Login Action__BMA-ULR.vi"("login info in"=w268) -> ("menu button action"=w274:string)
            n143 = call "Menu-Button Actions Acquisition(MainVI)__FP-BMA.vi"("error in (no error)"=w269, "event"=w274) -> ("error out"=w262:errorcluster)  [unwired: 7 in, 2 out]
          }
          frame True {
            n144 = call "Login Info FGV__BMA-ULR.vi"() -> ("login info out"=w278:T37)  [unwired: 2 in]
            n145 = call "Login Menu Button Properties Update__BMA-FP.vi"("login button"=w275, "menubar in"=w276, "login info in"=w278) -> ("error out"=w279:errorcluster, "login info out"=w282:T37)  [unwired: 7 in]
            n146 = call "Menu-Button Get User Login Action__BMA-ULR.vi"("login info in"=w282) -> ("menu button action"=w281:string)
            n147 = call "Menu-Button Actions Acquisition(MainVI)__FP-BMA.vi"("error in (no error)"=w279, "event"=w281) -> ("error out"=w280:errorcluster)  [unwired: 7 in, 2 out]
          }
        }
        n148 = Select(t="Macro: Exit", s=w253, f="") -> (s? t:f=w256:string)
        n149 = call "Add State(s) to Queue__jki_lib_state_machine.vi"("State(s) in Front (\"\")"=w256, "State(s) in (\"\")"=w261) -> ("States Out"=w260:string)  [unwired: 13 in]
      }
      frame "Users: Management" {
        # "/*弹出用户管理对话框*/"
        n150 = call "User Management__UM.vi"() -> ()  [unwired: 10 in]
        n151 = call "Add State(s) to Queue__jki_lib_state_machine.vi"("State(s) in (\"\")"=w286) -> ("States Out"=w285:string)  [unwired: 14 in]
      }
      frame "----------Event Proc File ----------" {
        # "/*分割线*/"
        n152 = call "Add State(s) to Queue__jki_lib_state_machine.vi"("State(s) in (\"\")"=w290) -> ("States Out"=w289:string)  [unwired: 14 in]
      }
      frame "File: Data Log" {
        # "/*添加功能VI！*/"
        # "/*用于处理事件记录*/"
        n153 = call "Add State(s) to Queue__jki_lib_state_machine.vi"("State(s) in (\"\")"=w294) -> ("States Out"=w293:string)  [unwired: 14 in]
      }
      frame "File: Copy Parameters" {
        # "/*添加功能VI！*/"
        # "/*用于处理复制参数*/"
        n154 = call "Add State(s) to Queue__jki_lib_state_machine.vi"("State(s) in (\"\")"=w298) -> ("States Out"=w297:string)  [unwired: 14 in]
      }
      frame "File: Print" {
        # "/*添加功能VI！*/"
        # "/*用于处理打印，打印内容未确定*/"
        n155 = call "Add State(s) to Queue__jki_lib_state_machine.vi"("State(s) in (\"\")"=w302) -> ("States Out"=w301:string)  [unwired: 14 in]
      }
      frame "File: Export" {
        # "/*添加功能VI！*/"
        # "/*处理导出文件*/"
        n156 = call "Add State(s) to Queue__jki_lib_state_machine.vi"("State(s) in (\"\")"=w306) -> ("States Out"=w305:string)  [unwired: 14 in]
      }
      frame "File: Exit" {
        # "/*响应退出*/"
        n157 = call "Add State(s) to Queue__jki_lib_state_machine.vi"("State(s) in Front (\"\")"="Macro: Exit" ("State(s) in Front (\"\")"), "State(s) in (\"\")"=w311) -> ("States Out"=w310:string)  [unwired: 13 in]
      }
      frame "----------Event Proc System ----------" {
        # "/*分割线*/"
        n158 = call "Add State(s) to Queue__jki_lib_state_machine.vi"("State(s) in (\"\")"=w315) -> ("States Out"=w314:string)  [unwired: 14 in]
      }
      frame "System: Comm Enable" {
        # "/*通信使能*/"
        # "/*添加功能VI！*/"
        n159 = call "Add State(s) to Queue__jki_lib_state_machine.vi"("State(s) in (\"\")"=w319) -> ("States Out"=w318:string)  [unwired: 14 in]
      }
      frame "System: Comm Disable" {
        # "/*添加功能VI！*/"
        # "/*通信禁用*/"
        n160 = call "Add State(s) to Queue__jki_lib_state_machine.vi"("State(s) in (\"\")"=w323) -> ("States Out"=w322:string)  [unwired: 14 in]
      }
      frame "System: Comm Diags" {
        # "/*添加功能VI！*/"
        # "/*通信诊断*/"
        n161 = Bundle By Name(cluster=w325, "Tab"=T9."通信诊断") -> (w324:T32)
        n162 = call "Add State(s) to Queue__jki_lib_state_machine.vi"("State(s) in (\"\")"=w329) -> ("States Out"=w328:string)  [unwired: 14 in]
      }
      frame "----------Event Proc Recipe ---------- " {
        # "/*分割线*/"
        n163 = call "Add State(s) to Queue__jki_lib_state_machine.vi"("State(s) in (\"\")"=w333) -> ("States Out"=w332:string)  [unwired: 14 in]
      }
      frame "Recipe: New" {
        # "/*添加功能VI！*/"
        # "/*新建Recipe*/"
        n164 = call "Add State(s) to Queue__jki_lib_state_machine.vi"("State(s) in (\"\")"=w337) -> ("States Out"=w336:string)  [unwired: 14 in]
      }
      frame "Recipe: Open" {
        # "/*添加功能VI！*/"
        # "/*打开Recipe*/"
        n165 = call "Add State(s) to Queue__jki_lib_state_machine.vi"("State(s) in (\"\")"=w341) -> ("States Out"=w340:string)  [unwired: 14 in]
      }
      frame "Recipe: Save" {
        # "/*添加功能VI！*/"
        # "/*保存Recipe*/"
        n166 = call "Add State(s) to Queue__jki_lib_state_machine.vi"("State(s) in (\"\")"=w345) -> ("States Out"=w344:string)  [unwired: 14 in]
      }
      frame "Recipe: Save As" {
        # "/*添加功能VI！*/"
        # "/*另存Recipe*/"
        n167 = call "Add State(s) to Queue__jki_lib_state_machine.vi"("State(s) in (\"\")"=w349) -> ("States Out"=w348:string)  [unwired: 14 in]
      }
      frame "Recipe: Remove" {
        # "/*添加功能VI！*/"
        # "/*删除Recipe*/"
        n168 = call "Add State(s) to Queue__jki_lib_state_machine.vi"("State(s) in (\"\")"=w353) -> ("States Out"=w352:string)  [unwired: 14 in]
      }
      frame "Recipe: Download" {
        # "/*添加功能VI！*/"
        # "/*下载Recipe*/"
        n169 = call "Add State(s) to Queue__jki_lib_state_machine.vi"("State(s) in (\"\")"=w357) -> ("States Out"=w356:string)  [unwired: 14 in]
      }
      frame "Recipe: Calendar" {
        # "/*添加功能VI！*/"
        # "/*Recipe的日历设置功能*/"
        n170 = Bundle By Name(cluster=w360, "Tab"=T9."设置时间信息") -> (w359:T32)
        n171 = call "Add State(s) to Queue__jki_lib_state_machine.vi"("State(s) in (\"\")"=w363) -> ("States Out"=w362:string)  [unwired: 14 in]
      }
      frame "Recipe: Time Builder" {
        # "/*添加功能VI！*/"
        # "/*Recipe的类型创建器功能*/"
        n172 = call "Add State(s) to Queue__jki_lib_state_machine.vi"("State(s) in (\"\")"=w367) -> ("States Out"=w366:string)  [unwired: 14 in]
      }
      frame "----------Event Proc EventLogs ---------- " {
        # "/*分割线*/"
        n173 = call "Add State(s) to Queue__jki_lib_state_machine.vi"("State(s) in (\"\")"=w371) -> ("States Out"=w370:string)  [unwired: 14 in]
      }
      frame "EventLogs: View" {
        # "/*响应按钮“查看事件记录”，从文本文件中读取所有发生过的事件。*/"
        n174 = call "EventLog Read__FS.vi"("error in (no error)"=w376) -> ("error out"=w375:errorcluster, "Event"=→"Event Strings":string)  [unwired: 9 in]
        n175 = Bundle By Name(cluster=w374, "Tab"=T9."查看事件记录") -> (w373:T32)
        n176 = call "Add State(s) to Queue__jki_lib_state_machine.vi"("State(s) in (\"\")"=w379) -> ("States Out"=w378:string)  [unwired: 14 in]
      }
      frame "EventLogs: Copy To A:" {
        # "/*添加功能VI！*/"
        # "/*将已发生过的事件复制到本地磁盘。*/"
        n177 = call "Add State(s) to Queue__jki_lib_state_machine.vi"("State(s) in (\"\")"=w383) -> ("States Out"=w382:string)  [unwired: 14 in]
      }
      frame "EventLogs: Remove" {
        # "/*添加功能VI！*/"
        # "/*删除部分已经发生的事件。*/"
        n178 = call "Add State(s) to Queue__jki_lib_state_machine.vi"("State(s) in (\"\")"=w387) -> ("States Out"=w386:string)  [unwired: 14 in]
      }
      frame "----------Event Proc Trend Plot ---------- " {
        # "/*添加功能VI！*/"
        # "/*分割线*/"
        n179 = call "Add State(s) to Queue__jki_lib_state_machine.vi"("State(s) in (\"\")"=w391) -> ("States Out"=w390:string)  [unwired: 14 in]
      }
      frame "TP: Graph" {
        # "/*添加功能VI！*/"
        # "/*实时观看当前的趋势图*/"
        n180 = control-ref of="Plot Scroll"() -> (w396:refnum<vi>)
        n181 = control-ref of="Plot Settings"() -> (w397:refnum<vi>)
        n182 = Bundle("Plot Settings"=w397, "Plot Scroll"=w396) -> (w395:T38)  [unwired: 1 in]
        n183 = Array Size(array="Plot Settings") -> ()  [unwired: 1 out]
        n184 = call "Scrollbar Index Array Set Properties__Uti.vi"("display rows (8)"=9, "array size"=10, "refnums"=w395) -> ()  [unwired: 8 in, 1 out]
        n185 = Bundle By Name(cluster=w400, "Tab"=T9."查看趋势图") -> (w399:T32)
        n186 = call "Add State(s) to Queue__jki_lib_state_machine.vi"("State(s) in (\"\")"=w403) -> ("States Out"=w402:string)  [unwired: 14 in]
      }
      frame "TP: Export Graph Data" {
        # "/*添加功能VI！*/"
        # "/*导出趋势图中的数据*/"
        n187 = call "Add State(s) to Queue__jki_lib_state_machine.vi"("State(s) in (\"\")"=w407) -> ("States Out"=w406:string)  [unwired: 14 in]
      }
      frame "----------Event Proc View ---------- " {
        # "/*分割线*/"
        n188 = call "Add State(s) to Queue__jki_lib_state_machine.vi"("State(s) in (\"\")"=w411) -> ("States Out"=w410:string)  [unwired: 14 in]
      }
      frame "View: Alarms" {
        # "/*添加功能VI！*/"
        # "/*查看警告*/"
        n189 = call "Add State(s) to Queue__jki_lib_state_machine.vi"("State(s) in (\"\")"=w415) -> ("States Out"=w414:string)  [unwired: 14 in]
      }
      frame "View: F4 Set up" {
        # "/*与F4进行单点数据交换*/"
        n190 = Cluster To Array(cluster="F4 Operation") -> (array=w425:T23[])
        n191 = call "File System Paths__FS.vi"() -> ("DynamicVIs"=w432:T39)  [unwired: 9 in, 2 out]
        n192 = Search 1D Array(1D array=w425, element=T22 TRUE ("元素")) -> (index of element=w429:i32)  [unwired: 1 in]
        n193 = Cluster To Array(cluster=w432) -> (array=w430:path[])
        n194 = Index Array(array=w430, index=w429) -> (element=w428:path)
        n195 = Open VI Reference(vi path=w428) -> (vi reference=w420:refnum<vi>, error out=w419:errorcluster)  [unwired: 5 in]
        n196 = call "Dynamic Call (Refnum)__Uti.vi"("error in (no error)"=w419, "open front panel? (T)"=FALSE, "vi reference in"=w420) -> ("error out"=w417:errorcluster, "vi reference out"=w418:refnum<vi>)  [unwired: 7 in]
        n197 = Bundle By Name(cluster=w422, "Tab"=T9."控制F4数据交换") -> (w424:T32)
        n198 = invoke on="子面板" class="子面板" method="Insert VI"(error in=w417, "VI Ref"=w418) -> (error out=w427:errorcluster)  [unwired: 2 in, 3 out]
        n199 = Close Reference(reference=w418, error in (no error)=w427) -> (error out=w421:errorcluster)
        n200 = call "Add State(s) to Queue__jki_lib_state_machine.vi"("State(s) in (\"\")"=w434) -> ("States Out"=w433:string)  [unwired: 14 in]
      }
      frame "View: Synergy Set up" {
        # "/*F4Profile编辑器，编辑Profile的工具*/"
        n201 = call "File System Paths__FS.vi"("error in (no error)"=w435) -> ("error out"=w437:errorcluster, "DynamicVIs"=w440:T39)  [unwired: 8 in, 1 out]
        n202 = Unbundle By Name(w440) -> ("Synergy Control"=w439:path)
        n203 = call "Dynamic Call__Uti.vi"("error in (no error)"=w437, "open front panel? (T)"=TRUE, "vi path"=w439) -> ("error out"=w436:errorcluster)  [unwired: 8 in]
        n204 = call "Add State(s) to Queue__jki_lib_state_machine.vi"("State(s) in (\"\")"=w443) -> ("States Out"=w442:string)  [unwired: 14 in]
      }
      frame "----------Event Proc Tools ---------- " {
        # "/*分割线*/"
        n205 = call "Add State(s) to Queue__jki_lib_state_machine.vi"("State(s) in (\"\")"=w447) -> ("States Out"=w446:string)  [unwired: 14 in]
      }
      frame "Tools: Set F4 Date and Time" {
        # "/*添加功能VI！*/"
        # "/*设置F4日期和时间*/"
        n206 = call "Add State(s) to Queue__jki_lib_state_machine.vi"("State(s) in (\"\")"=w451) -> ("States Out"=w450:string)  [unwired: 14 in]
      }
      frame "Tools: F4 Save Change to EE" {
        # "/*添加功能VI！*/"
        # "/*保存F4设置到EE？*/"
        n207 = call "Add State(s) to Queue__jki_lib_state_machine.vi"("State(s) in (\"\")"=w455) -> ("States Out"=w454:string)  [unwired: 14 in]
      }
      frame "Tools: F4 Profile Control" {
        # "/*F4Profile控制，下载已经编辑好的F4Profile至控制器上。*/"
        n208 = call "File System Paths__FS.vi"("error in (no error)"=w457) -> ("error out"=w458:errorcluster, "DynamicVIs"=w461:T39)  [unwired: 8 in, 1 out]
        n209 = Unbundle By Name(w461) -> ("Profile Control"=w460:path)
        n210 = call "Dynamic Call__Uti.vi"("error in (no error)"=w458, "open front panel? (T)"=TRUE, "vi path"=w460) -> ("error out"=w456:errorcluster)  [unwired: 8 in]
        n211 = call "Add State(s) to Queue__jki_lib_state_machine.vi"("State(s) in (\"\")"=w464) -> ("States Out"=w463:string)  [unwired: 14 in]
      }
      frame "Tools: F4 Profile Editor" {
        # "/*F4Profile编辑器，编辑Profile的工具*/"
        n212 = call "File System Paths__FS.vi"("error in (no error)"=w466) -> ("error out"=w468:errorcluster, "DynamicVIs"=w471:T39)  [unwired: 8 in, 1 out]
        n213 = Unbundle By Name(w471) -> ("Profile Editor"=w470:path)
        n214 = call "Dynamic Call__Uti.vi"("error in (no error)"=w468, "open front panel? (T)"=TRUE, "vi path"=w470) -> ("error out"=w467:errorcluster)  [unwired: 8 in]
        n215 = call "Add State(s) to Queue__jki_lib_state_machine.vi"("State(s) in Front (\"\")"="Macro: Exit" ("State(s) in Front (\"\")"), "State(s) in (\"\")"=w474) -> ("States Out"=w473:string)  [unwired: 13 in]
      }
    }
    n216 = Unbundle By Name(w71) -> ("Tab"=w70:T9)
    n217 = property on="Tab" class="TabCtl (strict)"("Value"=w70) -> ()  [unwired: 2 in, 2 out]
  }
